vi "Batch_ListBuildSpecProjects.vi"(8 "error in (no error)":errorcluster, 11 "CommandLine":string[](array[string])) -> (0 "error out":errorcluster, 2 "test details":string)   [LabVIEW 2019]
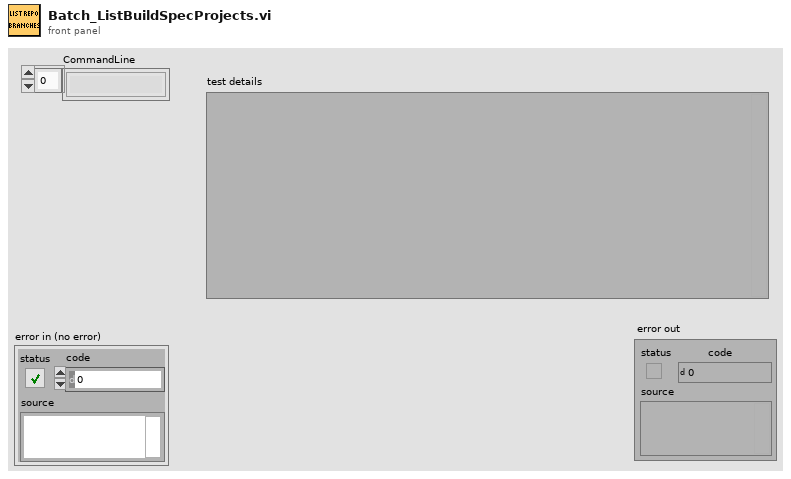
[diagram p1: front panel]
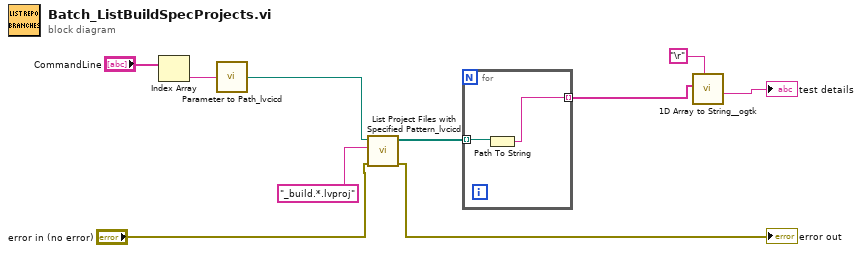
[diagram p0: block diagram]
diagram:
  n1 = Index Array(array="CommandLine") -> (element=w7:string)  [unwired: 1 in]
  n2 = call "Parameter to Path_lvcicd.vi"("String"=w7) -> ("Path"=w10:path)
  n3 = call "List Project Files with Specified Pattern_lvcicd.vi"("error in (no error)"="error in (no error)", "pattern"="_build.*.lvproj", "Path"=w10) -> ("error out"=→"error out":errorcluster, "All Files in Dir"=w3:path[])  [unwired: 6 in, 1 out]
  n4 = for {
    tunnel: w3 -> [w12] mode=indexing
    tunnel: [w11] -> w2 mode=indexing
    n5 = Path To String(path=w12) -> (string=w11:string)
  }
  n6 = call <userlib>:"1D Array to String__ogtk.vi"("delimiter (Tab)"="\r", "Array of Strings"=w2) -> ("delimited string"=→"test details":string)  [unwired: 9 in]
